vi "dger - General Matrix Rank-1 Update (DBL).vi"(6 "alpha":dbl=1.0, 9 "A":T1, 10 "y":dbl[](array[numeric]), 11 "x":dbl[](array[numeric])) -> (0 "error":i32, 3 "dger":T1)   [LabVIEW 2020, in "NI_AALBLAS.lvlib"]
doc: "Calculates the rank-1 update of a general matrix."
uses:
  NI_AALBLAS.lvlib
  RealMatrix.ctl
  Fucntion.ctl
  Order.ctl
  NI_Matrix.lvlib
panel:
  # "dger=alpha*x*y'+A"
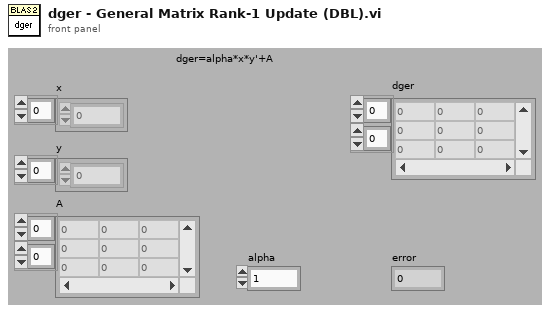
[diagram p1: front panel]
types:
  T1 = typedef "NI_Matrix.lvlib/RealMatrix.ctl" = dbl[][]
  T2 = typedef "NI_AALBLAS.lvlib/Order.ctl" = i32
  T3 = typedef "NI_AALBLAS.lvlib/Fucntion.ctl" = u16
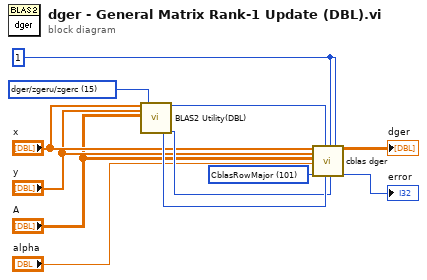
[diagram p0: block diagram]
diagram:
  w1 = 1
  w2 = T2 101 items=["CblasRowMajor"=101, "CblasColMajor"=102] ("order")
  w4 = T3 15 items=["ddot/zdotu/zdotc", "daxpy/zaxpy", "dnrm2/dznrm2", "dasum/dzasum", "dcopy/zcopy", "dswap/zswap", "drotm", "drot/zdrot", "idamax/izamax", "idamin/izamin", "dgemv/zgemv", "dsymv/zhemv", "dtrmv/ztrmv", "dsyr/zher", "dsyr2/zher2", "dger/zgeru/zgerc", "dtrsv/ztrsv", "dgemm/zgemm", "dsymm/zsymm/zhemm", "dtrmm/ztrmm", "dsyrk/zsyrk/zherk", "dsyr2k/zsyr2k/zher2k", "dtrsm/ztrsm"] ("function")
  n1 = call "BLAS2 Utility(DBL).vi"("x"="x", "y"="y", "A"="A", "function"=w4) -> ("m"=w12:i32, "lda"=w3:i32, "n"=w11:i32)  [unwired: 13 in]
  n2 = call "cblas dger.vi"("x"="x", "y"="y", "A"="A", "alpha"="alpha", "order"=w2, "lda"=w3, "m"=w12, "incx"=w1, "n"=w11, "incy"=w1) -> ("dger"=→"dger":T1, "error"=→"error":i32)  [unwired: 8 out]
